vi "navX Example (SPI - I2C).vi"() -> ()   [LabVIEW 2015]
uses:
  COMMON/TypeDefs/Value TypeDefs/navX Update Rate.ctl
  COMMON/TypeDefs/Data TypeDefs/navX Vector Data.ctl
  COMMON/TypeDefs/Data TypeDefs/navX YPRH Data.ctl
  COMMON/TypeDefs/Data TypeDefs/navX Quaternion Data.ctl
  COMMON/TypeDefs/Data TypeDefs/navX Status Data.ctl
  COMMON/TypeDefs/Value TypeDefs/navX NAVX_OP_STATUS.ctl
  COMMON/TypeDefs/Value TypeDefs/navX NAVX_CAL_STATUS.ctl
  COMMON/TypeDefs/Value TypeDefs/navX NAVX_SENSOR_STATUS.ctl
  COMMON/TypeDefs/Value TypeDefs/navX Interface Protocol.ctl
  COMMON/TypeDefs/Data TypeDefs/navX Board Information.ctl
  COMMON/TypeDefs/Value TypeDefs/navX NAVX_BOARD_CAPABILITY.ctl
  COMMON/TypeDefs/Value TypeDefs/navX NAVX_BOARD_YAW_AXIS.ctl
  <vilib>/Platform/TimedLoop/XDataNode/timing_clust.ctl
  <vilib>/Platform/TimedLoop/XDataNode/nitl_modes.ctl
  <vilib>/Platform/TimedLoop/XDataNode/wakeup.ctl
  <vilib>/platform/TimedLoop/XDataNode/XDataNode.xnode
  navX-MXP IMU.lvlib
  <vilib>/Platform/TimedLoop/XDataNode/XDNodeRunTimeDep.lvlib
panel:
  out "DISP x":dbl(graph)
  out "Disp Y":dbl(graph)
  out "Vel_Y":dbl(graph)
  out "Vel_X":dbl(graph)
  out "CRC Err Count":i32
  out "Board Information":T1
  in  "ZeroYaw":bool
  out "Velocity":T4
  out "Displacement":T4
  in  "Reset(F)":bool
  out "Timestamp":u32
  out "Fused Heading":dbl(knob) scale=0.0..360.0
  out "MPU Temperature (Centigrade)":dbl(slide) scale=20.0..40.0
  in  "navX Interface Protocol":T5
  out "Status":T6={"Update Rate Hz"=0, "Accelerometer Full-Scale Range"=0, "Gyro Full-Scale Range"=0, "NAVX_OP_STATUS"=0, "NAVX_CAL_STATUS"=0, "NAVX_SELFTEST_STATUS"=80, "NAVX_SENSOR_STATUS"={"MOVING"=FALSE, "YAW_STABLE"=FALSE, "MAG_DISTURBANCE"=FALSE, "ALTITUDE_VALID"=FALSE, "SEALEVEL_PRESS_SET"=FALSE, "FUSED_HEADING_VALID"=FALSE}} {"NAVX_OP_STATUS" items=["INITIALIZING", "SELFTEST_IN_PROGRESS", "ERROR", "IMU_AUTOCAL_IN_PROGRESS", "NORMAL"]; "NAVX_CAL_STATUS" items=["IMU_CAL_STATE_MASK"=3, "IMU_CAL_INPROGRESS"=0, "IMU_CAL_ACCUMULATE"=1, "IMU_CAL_COMPLETE"=2, "MAG_CAL_COMPLETE"=4, "BARO_CAL_COMPLETE"=8]}
  out "RawMag":T4
  out "RawGyro":T4
  out "RawAccel":T4
  out "Quaternion":T10
  out "YPRH":T11
  out "Acceleration":T4
  out "Valid?":bool
  in  "stop":bool
  out "Opened":bool
  in  "Update Rate (4Hz-60Hz)":T12=40 min=4 max=60 step=1
  # "SPI/I2C"
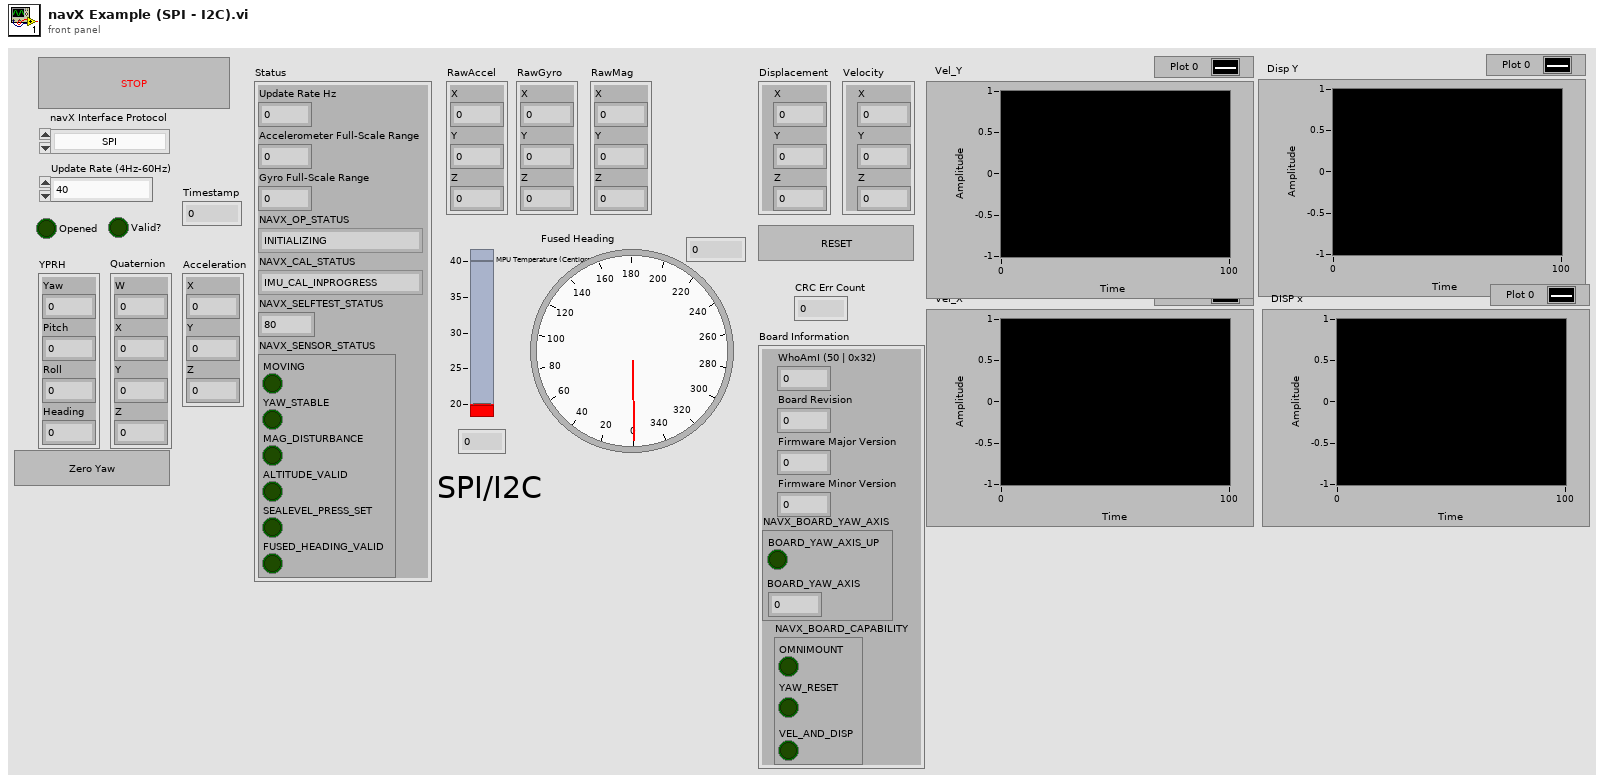
[diagram p1: front panel]
types:
  T1 = typedef "navX-MXP IMU.lvlib/navX Board Information.ctl" = cluster{"WhoAmI (50 | 0x32)":u8, "Board Revision":u8, "Firmware Major Version":u8, "Firmware Minor Version":u8, "NAVX_BOARD_CAPABILITY":T2, "NAVX_BOARD_YAW_AXIS":T3}
  T2 = typedef "navX-MXP IMU.lvlib/navX NAVX_BOARD_CAPABILITY.ctl" = cluster{"OMNIMOUNT":bool, "YAW_RESET":bool, "VEL_AND_DISP":bool}
  T3 = typedef "navX-MXP IMU.lvlib/navX NAVX_BOARD_YAW_AXIS.ctl" = cluster{"BOARD_YAW_AXIS_UP":bool, "BOARD_YAW_AXIS":u8}
  T4 = typedef "navX-MXP IMU.lvlib/navX Vector Data.ctl" = cluster{"X":dbl, "Y":dbl, "Z":dbl}
  T5 = typedef "navX-MXP IMU.lvlib/navX Interface Protocol.ctl" = enum16{"SPI", "I2C", "SERIAL"}
  T6 = typedef "navX-MXP IMU.lvlib/navX Status Data.ctl" = cluster{"Update Rate Hz":u8, "Accelerometer Full-Scale Range":u8, "Gyro Full-Scale Range":u16, "NAVX_OP_STATUS":T7, "NAVX_CAL_STATUS":T8, "NAVX_SELFTEST_STATUS":u8, "NAVX_SENSOR_STATUS":T9}
  T7 = typedef "navX-MXP IMU.lvlib/navX NAVX_OP_STATUS.ctl" = u8
  T8 = typedef "navX-MXP IMU.lvlib/navX NAVX_CAL_STATUS.ctl" = u8
  T9 = typedef "navX-MXP IMU.lvlib/navX NAVX_SENSOR_STATUS.ctl" = cluster{"MOVING":bool, "YAW_STABLE":bool, "MAG_DISTURBANCE":bool, "ALTITUDE_VALID":bool, "SEALEVEL_PRESS_SET":bool, "FUSED_HEADING_VALID":bool}
  T10 = typedef "navX-MXP IMU.lvlib/navX Quaternion Data.ctl" = cluster{"W":dbl, "X":dbl, "Y":dbl, "Z":dbl}
  T11 = typedef "navX-MXP IMU.lvlib/navX YPRH Data.ctl" = cluster{"Yaw":dbl, "Pitch":dbl, "Roll":dbl, "Heading":dbl}
  T12 = typedef "navX-MXP IMU.lvlib/navX Update Rate.ctl" = u8
  T13 = typedef "navX-MXP IMU.lvlib/navX Device TypeDef.ctl" = cluster{"navX Interface Protocol":T5, "navX Interface Protocol TypeDefs":cluster{"SPIDevRef":T14, "I2CDevRef":T16}, "navX System Information":cluster{"Board Information":T1, "Status":T6, "Offsets":T18, "LastSampleTimestamp":dbl, "LastSampleValid":bool}, "navX Common Information":cluster{"Update Rate (4Hz-60Hz)":T12, "refnum name":string, "error":errorcluster, "LastSampleFPGATimestamp":dbl}}
  T14 = typedef "WPI_SPIDevRef.ctl" = cluster{"DevStatus":errorcluster, "Handle":i32, "SPI Bus":T15}
  T15 = typedef "spi_bus.ctl" = enum16{"SPI On-Board, CS0", "SPI On-Board, CS1", "SPI On-Board, CS2", "SPI On-Board, CS3", "SPI MXP", "Invalid"}
  T16 = typedef "WPI_I2CDevRef.ctl" = cluster{"DevStatus":errorcluster, "Device Address":u8, "Handle":i32, "I2C Bus":T17}
  T17 = typedef "i2c_bus.ctl" = enum16{"I2C On-Board", "I2C MXP", "Invalid"}
  T18 = typedef "navX-MXP IMU.lvlib/navX Offsets Data.ctl" = cluster{"Yaw":dbl, "Quat W":dbl, "Quat X":dbl, "Quat Y":dbl, "Quat Z":dbl}
  T19 = typedef "XDNodeRunTimeDep.lvlib/timing_clust.ctl" = cluster{"Expected End [f-1]":u64, "Actual End [f-1]":u64, "Finished Late? [f-1]":bool, "Expected End [i-1]":u64, "Actual End [i-1]":u64, "Finished Late? [i-1]":bool, "Expected Start [i]":u64, "Actual Start [i]":u64, "Expected Start [f]":u64, "Actual Start [f]":u64, "Source Name":string, "Structure Name":string, "Period":i64, "Deadline":i64, "Offset":i64, "Start":i64, "Priority":i32, "Timeout":i32, "Mode":T20, "Wakeup Reason":T21, "Error":errorcluster, "Source Type":string, "Secondary Source Type":string, "Global End Time":u64, "Global Start Time":u64, "Frame Duration":u64, "Iteration Duration":u64, "Assigned CPU":i32, "I/O Scan Engine Mode":u32}
  T20 = typedef "XDNodeRunTimeDep.lvlib/nitl_modes.ctl" = enum32{"No Change", "Process missed periods, maintain original phase", "Discard missed periods, maintain original phase", "Process missed periods, ignore original phase", "Discard missed periods, ignore original phase"}
  T21 = typedef "XDNodeRunTimeDep.lvlib/wakeup.ctl" = enum32{"Normal", "Aborted", "Asynchronous wakeup", "Timing source error", "Timed loop error", "Timeout"}
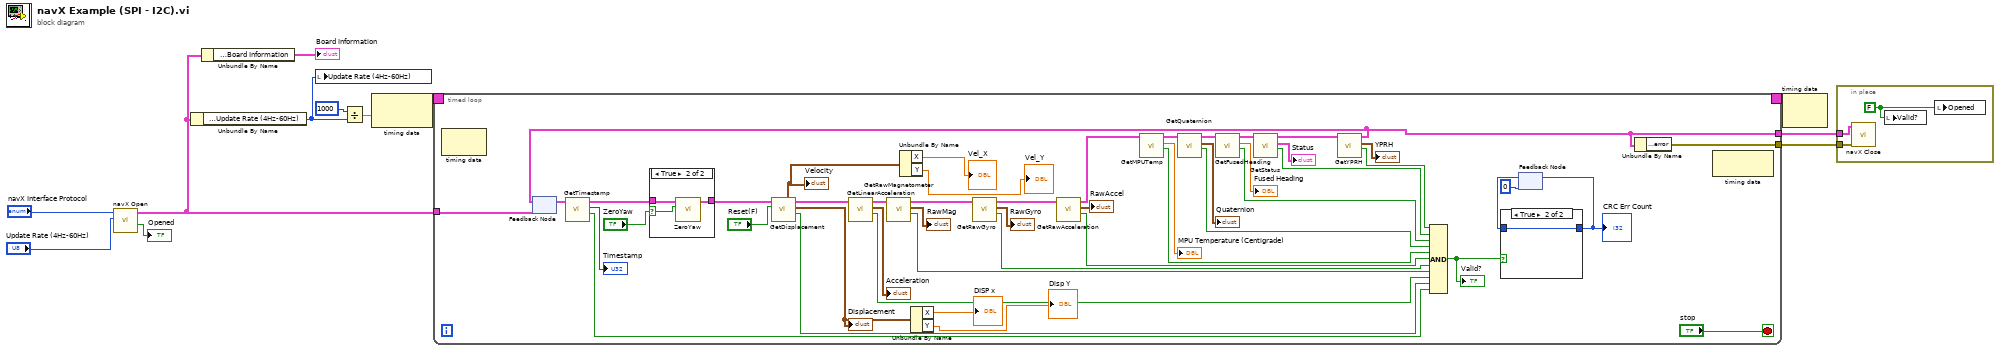
[diagram p0: block diagram]
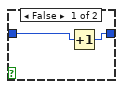
[diagram p2: hidden frame]
diagram:
  n1 = call "navX Open.vi"("Update Rate (4Hz-60Hz)"="Update Rate (4Hz-60Hz)", "navX Interface Protocol"="navX Interface Protocol") -> ("Opened?"=→"Opened":bool, "navX Device TypeDef"=w2:T13)  [unwired: 7 in, 1 out]
  n2 = Unbundle By Name(w2) -> ("navX Common Information.Update Rate (4Hz-60Hz)"=w8:T12)
  n3 = Unbundle By Name(w2) -> ("navX System Information.Board Information"=→"Board Information":T1)
  n4 = local write "Update Rate (4Hz-60Hz)"(w8) -> ()
  n5 = Divide(x=1000, y=w8) -> (x/y=w5:dbl)
  n6 = node-c288(w5) -> (w7:T19)
  n7 = timed-loop {
    timing: w7 -> [_]
    timing-out: [_] -> w6
    tunnel: w2 -> [w23]
    tunnel: [w21] -> w3
    tunnel: [w58] -> w4
    stop <- "stop" stop-if-true
    n8 = node-c288() -> ()  [unwired: 1 in, 1 out]
    n9 = feedback #1(w23) -> (w22:T13)
    n10 = call "GetTimestamp.vi"("navX Device TypeDef"=w22) -> ("Valid?"=w32:bool, "Timestamp"=→"Timestamp":u32, "navX Device TypeDef"=w29:T13)  [unwired: 8 in]
    n11 = case shown="True" "ZeroYaw" {
      selector: "ZeroYaw" -> [_ w66]
      tunnel: w29 -> [w65 w68]
      tunnel: [w65 w67] -> w28
      frame False {
      }
      frame True {
        n12 = call "ZeroYaw.vi"("Reset(F)"=w66, "navX Device TypeDef"=w68) -> ("navX Device TypeDef"=w67:T13)  [unwired: 8 in, 1 out]
      }
    }
    n13 = call "GetDisplacement.vi"("Reset(F)"="Reset(F)", "navX Device TypeDef"=w28) -> ("Valid?"=w31:bool, "Displacement"=w15:T4, "navX Device TypeDef 2"=w33:T13, "Velocity"=w18:T4)  [unwired: 6 in]
    "Displacement" <- w15
    "Velocity" <- w18
    n14 = call "GetLinearAcceleration.vi"("navX Device TypeDef"=w33) -> ("Valid?"=w36:bool, "Linear Acceleration"=→"Acceleration":T4, "navX Device TypeDef"=w37:T13)  [unwired: 8 in]
    n15 = call "GetRawMagnetometer.vi"("navX Device TypeDef"=w37) -> ("Valid?"=w38:bool, "Raw Magnetometer"=→"RawMag":T4, "navX Device TypeDef"=w40:T13)  [unwired: 8 in]
    n16 = Unbundle By Name(w18) -> ("X"=→"Vel_X":dbl, "Y"=→"Vel_Y":dbl)
    n17 = Unbundle By Name(w15) -> ("X"=→"DISP x":dbl, "Y"=→"Disp Y":dbl)
    n18 = call "GetRawGyro.vi"("navX Device TypeDef"=w40) -> ("Valid?"=w41:bool, "Raw Gyro"=→"RawGyro":T4, "navX Device TypeDef"=w43:T13)  [unwired: 8 in]
    n19 = call "GetRawAcceleration.vi"("navX Device TypeDef"=w43) -> ("Valid?"=w44:bool, "Raw Acceleration"=→"RawAccel":T4, "navX Device TypeDef"=w46:T13)  [unwired: 8 in]
    n20 = call "GetMPUTemp.vi"("navX Device TypeDef"=w46) -> ("Valid?"=w47:bool, "MPU Temperature (Centigrade)"=→"MPU Temperature (Centigrade)":dbl, "navX Device TypeDef"=w49:T13)  [unwired: 8 in]
    n21 = call "GetQuaternion.vi"("navX Device TypeDef"=w49) -> ("Valid?"=w51:bool, "Quaternion"=→"Quaternion":T10, "navX Device TypeDef"=w52:T13)  [unwired: 8 in]
    n22 = call "GetFusedHeading.vi"("navX Device TypeDef"=w52) -> ("Valid?"=w53:bool, "Fused Heading"=→"Fused Heading":dbl, "navX Device TypeDef"=w54:T13)  [unwired: 8 in]
    n23 = call "GetStatus.vi"("navX Device TypeDef"=w54) -> ("Valid?"=w55:bool, "Status"=→"Status":T6, "navX Device TypeDef"=w57:T13)  [unwired: 8 in]
    n24 = call "GetYPRH.vi"("navX Device TypeDef"=w57) -> ("Valid?"=w60:bool, "YPRH"=→"YPRH":T11, "navX Device TypeDef"=w21:T13)  [unwired: 8 in]
    n25 = feedback-in #1(w21) -> ()
    n26 = Compound Arithmetic op=AND(w60, w55, w53, w51, w47, w44, w41, w38, w36, w31, w32) -> (w24:bool)
    "Valid?" <- w24
    n27 = feedback #2(0) -> (w25:i32)
    n28 = case shown="True" w24 {
      tunnel: w25 -> [w63 w64]
      tunnel: [w62 w64] -> w27
      frame False {
        n29 = Increment(x=w63) -> (x+1=w62:i32)
      }
      frame True {
      }
    }
    "CRC Err Count" <- w27
    n30 = feedback-in #2(w27) -> ()
    n31 = Unbundle By Name(w21) -> ("navX Common Information.error"=w58:errorcluster)
    n32 = node-c288() -> ()  [unwired: 1 in, 1 out]
  }
  n33 = node-c288(w6) -> ()  [unwired: 1 out]
  n34 = in-place {
    in-place-border: w3 -> [w73]
    in-place-border: w4 -> [w72]
    w71 = FALSE ("Valid?")
    n35 = call "navX Close.vi"("error in (no error)"=w72, "navX Device TypeDef"=w73) -> ()  [unwired: 9 in, 1 out]
    n36 = local write "Valid?"(w71) -> ()
    n37 = local write "Opened"(w71) -> ()
  }
